vi "Parse API JSON Response.vi"(8 "error in":errorcluster, 11 "API Response":string) -> (0 "error out":errorcluster, 3 "Weather Forecast Data":T1)   [LabVIEW 2025, in "Weather Actor.lvlib" / "Weather.lvclass"]
uses:
  Weather.lvclass
  Weather.lvclass/Weather.ctl
  <vilib>/addons/_JKI.lib/Serialization/JSON/JKI JSON Serialization.lvlib
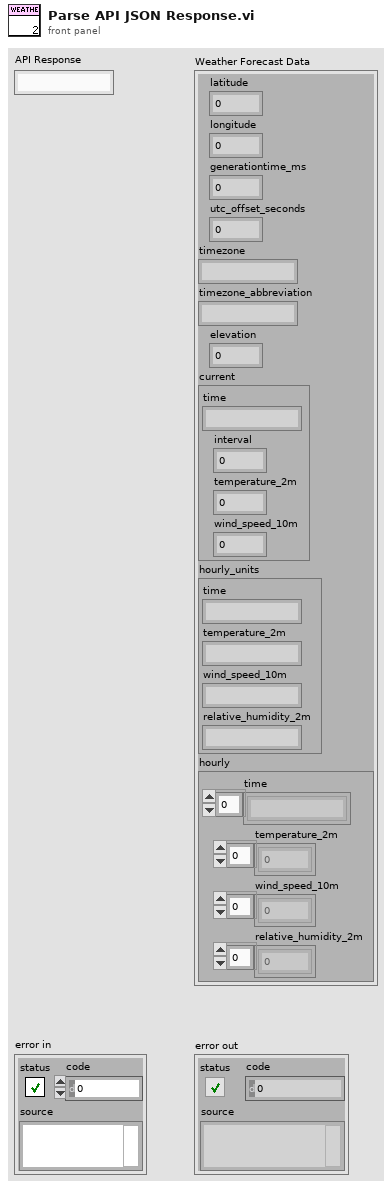
[diagram p1: front panel]
types:
  T1 = cluster{"latitude":dbl, "longitude":dbl, "generationtime_ms":dbl, "utc_offset_seconds":i32, "timezone":string, "timezone_abbreviation":string, "elevation":dbl, "current":cluster{"time":string, "interval":i32, "temperature_2m":dbl, "wind_speed_10m":dbl}, "hourly_units":cluster{"time":string, "temperature_2m":string, "wind_speed_10m":string, "relative_humidity_2m":string}, "hourly":cluster{"time":string[], "temperature_2m":dbl[], "wind_speed_10m":dbl[], "relative_humidity_2m":dbl[]}}
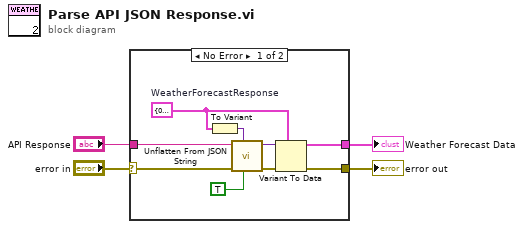
[diagram p0: block diagram]
diagram:
  n1 = case shown="No Error" "error in" {
    selector: "error in" -> [w8 w14]
    tunnel: [w7 w14] -> w3
    tunnel: [w6 _] -> w2
    tunnel: "API Response" -> [w5 _]
    frame No Error {
      w13 = T1 {"latitude"=0.0, "longitude"=0.0, "generationtime_ms"=0.0, "utc_offset_seconds"=0, "timezone"="", "timezone_abbreviation"="", "elevation"=0.0, "current"={"time"="", "interval"=0, "temperature_2m"=0.0, "wind_speed_10m"=0.0}, "hourly_units"={"time"="", "temperature_2m"="", "wind_speed_10m"="", "relative_humidity_2m"=""}, "hourly"={"time"=[], "temperature_2m"=[], "wind_speed_10m"=[], "relative_humidity_2m"=[]}}  # WeatherForecastResponse
      n2 = To Variant(anything=w13) -> (Variant=w12:variant)
      n3 = call <vilib>:"Unflatten From JSON String.vi"("Nulls as Defaults (F)"=TRUE, "Type and Defaults"=w12, "error in"=w8, "JSON String"=w5) -> ("error out"=w11:errorcluster, "Variant"=w10:variant)  [unwired: 6 in]
      n4 = Variant To Data(error in=w11, type=w13, Variant=w10) -> (data=w6:T1, error out=w7:errorcluster)
    }
    frame Error {
    }
  }
  "error out" <- w3
  "Weather Forecast Data" <- w2
